vi "control pwm host.vi"() -> ()   [LabVIEW 2023]
panel:
  out "PWM":dbl(knob) scale=0.0..100.0
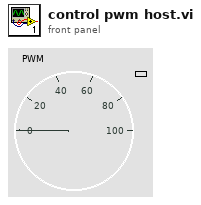
[diagram p1: front panel]
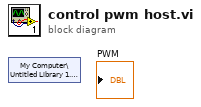
[diagram p0: block diagram]
diagram:
  n1 = shared-variable "My Computer\\Untitled Library 1.lvlib\\PWM"() -> ()  [unwired: 1 in, 2 out]
